vi "UT1_E3_ContadorFlancos.vi"() -> ()   [LabVIEW 2024]
panel:
  out "Contador":dbl
  in  "stop":bool
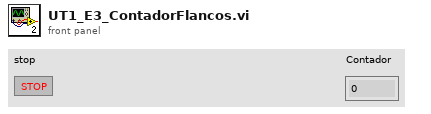
[diagram p1: front panel]
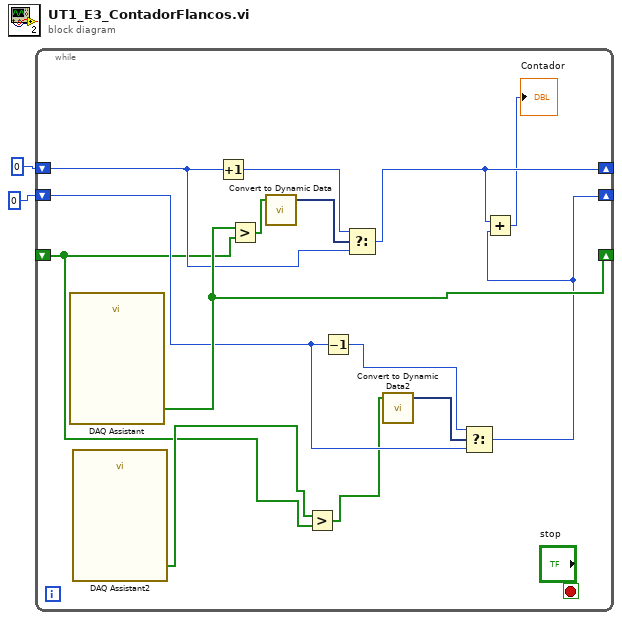
[diagram p0: block diagram]
diagram:
  n1 = while {
    shift-right: [w5] -> _
    shift-left: 0 -> [w10]
    shift-right: [w11] -> _
    shift-left: _ -> [w6]
    shift-right: [w4] -> _
    shift-left: 0 -> [w9]
    stop <- "stop" stop-if-true
    n2 = call "DAQ Assistant"() -> ("data"=w11:bool[])  [unwired: 17 in, 2 out]
    n3 = call "DAQ Assistant2"() -> ("data"=w7:bool[])  [unwired: 17 in, 2 out]
    n4 = Increment(x=w10) -> (x+1=w16:i32)
    n5 = Greater?(x=w11, y=w6) -> (0:w15:bool[])
    n6 = call "Convert to Dynamic Data"("Array"=w15) -> ("Dynamic Data Type"=w14:dynamicdata)  [unwired: 3 in]
    n7 = Greater?(x=w7, y=w6) -> (0:w8:bool[])
    n8 = Decrement(x=w9) -> (x-1=w12:i32)
    n9 = Select(t=w16, s=w14, f=w10) -> (s? t:f=w5:i32)
    n10 = call "Convert to Dynamic Data2"("Array"=w8) -> ("Dynamic Data Type"=w13:dynamicdata)  [unwired: 3 in]
    n11 = Select(t=w12, s=w13, f=w9) -> (s? t:f=w4:i32)
    n12 = Add(x=w5, y=w4) -> (x+y=→"Contador":i32)
  }
